vi "Write SerialNo.vi"(8 "error in (no error)":errorcluster, 10 "SerialNo":string, 11 "Monochromator in":refnum<class "Monochromator.lvclass">) -> (0 "error out":errorcluster, 3 "Monochromator out":refnum<class "Monochromator.lvclass">)   [LabVIEW 2023, in "Monochromator.lvclass"]
uses:
  Monochromator.lvclass
  GenericDevice/GenericDevice.lvclass
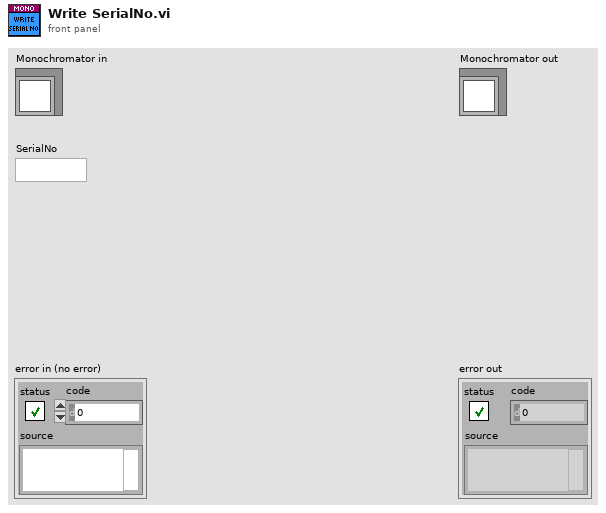
[diagram p1: front panel]
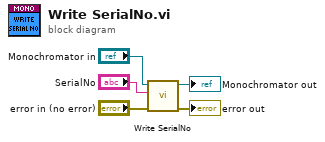
[diagram p0: block diagram]
diagram:
  n1 = call-parent "Write SerialNo.vi"("error in (no error)"="error in (no error)", "SerialNo"="SerialNo", "GenericDevice in"="Monochromator in") -> ("error out"=→"error out":errorcluster, "GenericDevice out"=→"Monochromator out":refnum<class "Monochromator.lvclass">)  [unwired: 7 in]
